vi "Publish Stats.vi"(8 "error in (no error)":errorcluster, 11 "System Health Module in":refnum<class "System Health Module.lvclass">) -> (0 "error out":errorcluster, 3 "System Health Module out":refnum<class "System Health Module.lvclass">)   [LabVIEW 2020, in "Volatus.lvlib" / "System Health Module.lvclass"]
uses:
  System Health Module.lvclass
  C:/dev/lv20CE/relink/lv-volatus/Volatus/Module/Module.lvclass
  System Health Module.lvclass/System Health Module.ctl
  Module/Module.lvclass/Module.ctl
  VolatusAPI/VolatusAPI.lvclass/VolatusAPI.ctl
  lv-vecto/Vecto/Group/Group.lvclass
  C:/dev/lv20CE/relink/lv-vecto/Vecto/GroupAbstract/GroupAbstract.lvclass
  System SAL/System SAL.lvclass
  Module/Module.lvclass
  C:/dev/lv20CE/relink/lv-volatus/Volatus/System Health Module/System Health Module.lvclass
  C:/dev/lv20CE/relink/lv-vecto/Vecto/Group/Group.lvclass
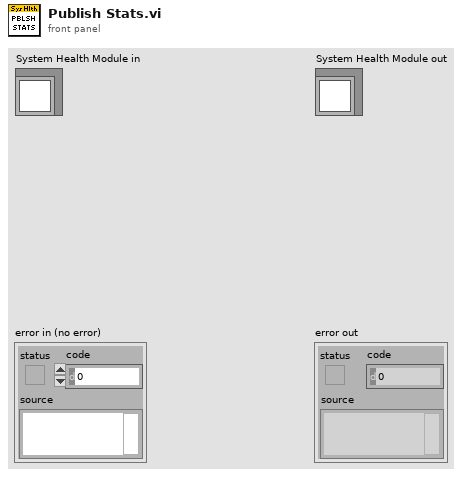
[diagram p1: front panel]
types:
  T1 = typedef "Volatus.lvlib/System Health Module.lvclass/Drive Info.ctl" = cluster{"Config":T2, "Capacity GB":dbl, "Used GB":dbl, "Next Warning":dbl, "Next Error":dbl}
  T2 = typedef "Volatus.lvlib/System Health Module.lvclass/Drive Config.ctl" = cluster{"Path":path, "Warning GB":dbl, "Error GB":dbl}
  T3 = typedef "Volatus.lvlib/System SAL.lvclass/Performance Values.ctl" = cluster{"CPU Total %":dbl, "Mem Avail GB":dbl, "Mem Free GB":dbl}
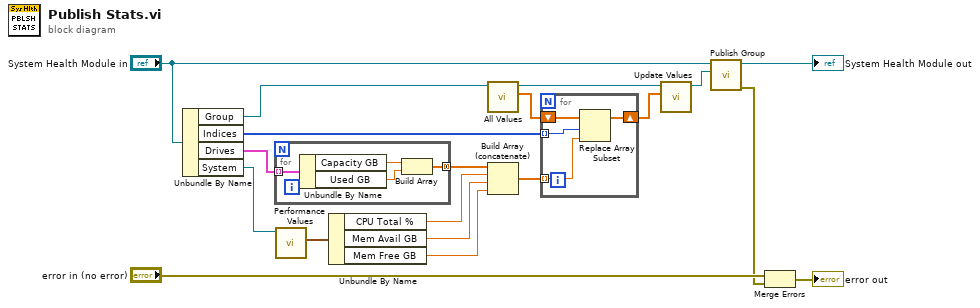
[diagram p0: block diagram]
diagram:
  n1 = Unbundle By Name("System Health Module in") -> ("Group"=w4:refnum<class "Group.lvclass">, "Indices"=w10:i32[], "Drives"=w17:T1[], "System"=w15:refnum<class "System SAL.lvclass">)
  n2 = for {
    tunnel: w17 -> [w23] mode=indexing
    tunnel: [w20] -> w16 mode=concatenating
    n3 = Unbundle By Name(w23) -> ("Capacity GB"=w22:dbl, "Used GB"=w21:dbl)
    n4 = Build Array(w22, w21) -> (w20:dbl[])
  }
  n5 = call-dynamic "Performance Values.vi"("System SAL in"=w15) -> ("Performance Values"=w14:T3)  [unwired: 9 in, 1 out]
  n6 = Unbundle By Name(w14) -> ("CPU Total %"=w13:dbl, "Mem Avail GB"=w12:dbl, "Mem Free GB"=w11:dbl)
  n7 = call "All Values.vi"("Group in"=w4) -> ("Scaled"=w2:dbl[], "Group out"=w3:refnum<class "Group.lvclass">)  [unwired: 6 in, 3 out]
  n8 = Build Array (concatenate)(w16, w13, w12, w11) -> (w9:dbl[])
  n9 = for {
    tunnel: w10 -> [w26] mode=indexing
    tunnel: w9 -> [w25] mode=indexing
    shift-right: [w24] -> w1
    shift-left: w2 -> [w27]
    n10 = Replace Array Subset(array=w27, new element=w25, index=w26) -> (w24:dbl[])
  }
  n11 = call "Update Values.vi"("Values"=w1, "Group in"=w3) -> ("Group out"=w7:refnum<class "Group.lvclass">)  [unwired: 8 in, 1 out]
  n12 = call "Publish Group.vi"("Group"=w7, "Module in"="System Health Module in") -> ("error out"=w5:errorcluster, "Module out"=→"System Health Module out":refnum<class "System Health Module.lvclass">)  [unwired: 8 in]
  n13 = Merge Errors("error in (no error)", w5) -> (→"error out":errorcluster)
